vi "Probador de cables TEST.vi"() -> ()   [LabVIEW 2013]
doc: "This example performs a serial port write and a serial port read. The parameters set for the serial port must match the parameters of the connected instrument or device. The VISA Configure Serial Port VI sets the configuration parameters. The front panel displays the controls used to configure the basic parameters, such as baud rate, data bits, and parity. The VI passes the VISA resource name to other VIs that perform operations on that VISA resource. The VISA Write function sends a command to the serial device and the VISA Read function returns data based on the command. The VISA Close function then closes the reference to the serial device. It is important to close the reference; otherwise, further communication through that port might not be possible."
uses:
  <vilib>/Platform/TimedLoop/XDataNode/timing_clust.ctl
  <vilib>/Platform/TimedLoop/XDataNode/nitl_modes.ctl
  <vilib>/Platform/TimedLoop/XDataNode/wakeup.ctl
  <vilib>/Instr/_visa.llb/VISA Configure Serial Port (Instr).vi
  <vilib>/platform/TimedLoop/XDataNode/XDataNode.xnode
  <vilib>/Platform/TimedLoop/XDataNode/XDNodeRunTimeDep.lvlib
panel:
  out "Serial Settings:Number of Bytes at Serial Port 2":u32
  out "in":u8[](array[numeric])
  out "Serial Settings:Number of Bytes at Serial Port":u32
  out "OK?":bool
  out "out":u8[](array[numeric])
  in  "Send":bool
  in  "Pin":u8
  in  "stop":bool
  in  "VISA resource name":refnum<visa-resource-name>="COM1"
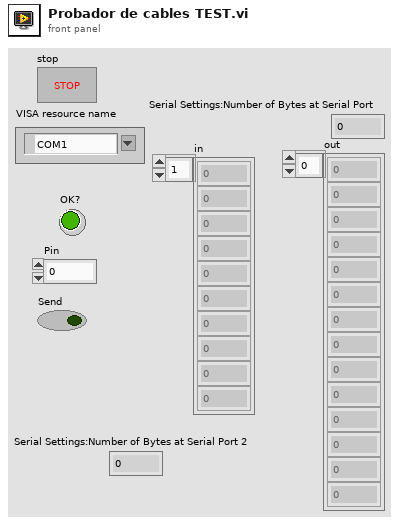
[diagram p1: front panel]
types:
  T1 = typedef "XDNodeRunTimeDep.lvlib/timing_clust.ctl" = cluster{"Expected End [f-1]":u64, "Actual End [f-1]":u64, "Finished Late? [f-1]":bool, "Expected End [i-1]":u64, "Actual End [i-1]":u64, "Finished Late? [i-1]":bool, "Expected Start [i]":u64, "Actual Start [i]":u64, "Expected Start [f]":u64, "Actual Start [f]":u64, "Source Name":string, "Structure Name":string, "Period":i64, "Deadline":i64, "Offset":i64, "Start":i64, "Priority":i32, "Timeout":i32, "Mode":T2, "Wakeup Reason":T3, "Error":errorcluster, "Source Type":string, "Secondary Source Type":string, "Global End Time":u64, "Global Start Time":u64, "Frame Duration":u64, "Iteration Duration":u64, "Assigned CPU":i32, "I/O Scan Engine Mode":u32}
  T2 = typedef "XDNodeRunTimeDep.lvlib/nitl_modes.ctl" = enum32{"No Change", "Process missed periods, maintain original phase", "Discard missed periods, maintain original phase", "Process missed periods, ignore original phase", "Discard missed periods, ignore original phase"}
  T3 = typedef "XDNodeRunTimeDep.lvlib/wakeup.ctl" = enum32{"Normal", "Aborted", "Asynchronous wakeup", "Timing source error", "Timed loop error", "Timeout"}
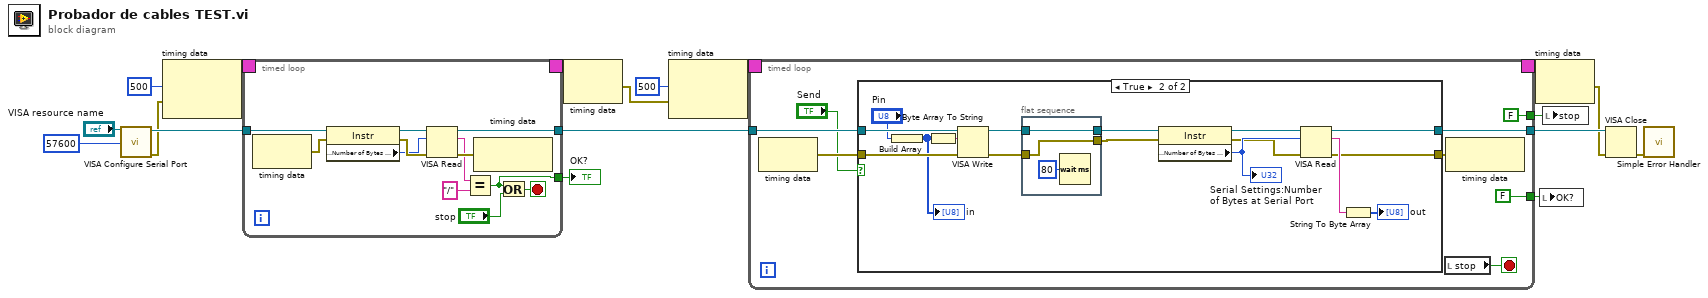
[diagram p0: block diagram]
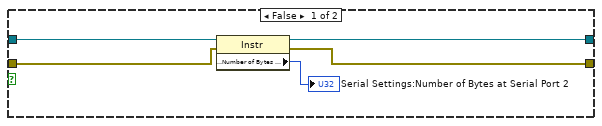
[diagram p2: hidden frame]
diagram:
  n1 = call-poly "VISA Configure Serial Port"("VISA resource name"="VISA resource name", "baud rate (9600)"=u32 57600) -> ("VISA resource name out"=w17:refnum<visa-resource-name>, "error out"=w14:errorcluster)  [unwired: 7 in, 5 out]
  n2 = node-c288(i64 500 ("Period"), w14) -> (w16:T1)
  n3 = timed-loop {
    timing: w16 -> [_]
    timing-out: [_] -> w15
    tunnel: [w30] -> w4
    tunnel: w17 -> [w29]
    tunnel: [w19] -> w7
    stop <- w20 stop-if-true
    n4 = node-c288() -> (w25:errorcluster)  [unwired: 1 in]
    n5 = property class="Instr"(reference=w29, error in=w25) -> (reference out=w28:refnum<visa-resource-name>, error out=w27:errorcluster, "Serial Settings:Number of Bytes at Serial Port"=w26:u32)
    n6 = VISA Read(VISA resource name=w28, byte count=w26, error in (no error)=w27) -> (VISA resource name out=w30:refnum<visa-resource-name>, read buffer=w23:string, error out=w24:errorcluster)  [unwired: 1 out]
    n7 = Equal?(x=w23, y="/") -> (x = y?=w19:bool)
    n8 = node-c288(w24) -> ()  [unwired: 1 out]
    n9 = Or(x=w19, y="stop") -> (x .or. y?=w20:bool)
  }
  "OK?" <- w7
  n10 = node-c288(w15) -> (w3:errorcluster)
  n11 = node-c288(i64 500 ("Period"), w3) -> (w10:T1)
  n12 = timed-loop {
    timing: w10 -> [_]
    timing-out: [_] -> w9
    tunnel: w4 -> [w43]
    tunnel: [FALSE ("stop")] -> w11
    tunnel: [w41] -> w2
    tunnel: [FALSE ("OK?")] -> w6
    stop <- w40 stop-if-true
    n13 = node-c288() -> (w39:errorcluster)  [unwired: 1 in]
    n14 = case shown="True" "Send" {
      tunnel: w43 -> [w47 w64]
      tunnel: [w44 w62] -> w41
      tunnel: w39 -> [w46 w61]
      tunnel: [w45 w60] -> w38
      frame False {
        n15 = property class="Instr"(reference=w47, error in=w46) -> (reference out=w44:refnum<visa-resource-name>, error out=w45:errorcluster, "Serial Settings:Number of Bytes at Serial Port"=→"Serial Settings:Number of Bytes at Serial Port 2":u32)
      }
      frame True {
        n16 = Build Array("Pin") -> (w53:u8[])
        "in" <- w53
        n17 = Byte Array To String ("Byte Array \nTo String")(unsigned byte array=w53) -> (string=w58:string)
        n18 = VISA Write(VISA resource name=w64, write buffer=w58, error in (no error)=w61) -> (VISA resource name out=w52:refnum<visa-resource-name>, error out=w51:errorcluster)  [unwired: 1 out]
        n19 = flat-sequence {
          tunnel: w52 -> [w67]
          tunnel: w51 -> [w66]
          tunnel: [w67] -> w50
          tunnel: [w66] -> w49
          frame #0 {
            n20 = Wait (ms)(milliseconds to wait=u32 80) -> ()  [unwired: 1 out]
          }
        }
        n21 = property class="Instr"(reference=w50, error in=w49) -> (reference out=w56:refnum<visa-resource-name>, error out=w54:errorcluster, "Serial Settings:Number of Bytes at Serial Port"=w55:u32)
        "Serial Settings:Number of Bytes at Serial Port" <- w55
        n22 = VISA Read(VISA resource name=w56, byte count=w55, error in (no error)=w54) -> (VISA resource name out=w62:refnum<visa-resource-name>, read buffer=w63:string, error out=w60:errorcluster)  [unwired: 1 out]
        n23 = String To Byte Array(string=w63) -> (unsigned byte array=→"out":u8[])
      }
    }
    n24 = local read "stop"() -> (w40:bool)
    n25 = node-c288(w38) -> ()  [unwired: 1 out]
  }
  n26 = node-c288(w9) -> (w1:errorcluster)
  n27 = local write "OK?"(w6) -> ()
  n28 = local write "stop"(w11) -> ()
  n29 = VISA Close(VISA resource name=w2, error in (no error)=w1) -> (error out=w12:errorcluster)
  n30 = call <vilib>:"Simple Error Handler.vi"("error in (no error)"=w12) -> ()  [unwired: 4 in, 5 out]
